vi "Write SA Pin.vi"(8 "error in (no error)":errorcluster, 10 "SA Pin":string, 11 "TDSCDMA_MODACC in":refnum<class "TDSCDMA_MODACC.lvclass">=refnum) -> (0 "error out":errorcluster, 3 "TDSCDMA_MODACC out":refnum<class "TDSCDMA_MODACC.lvclass">)   [LabVIEW 2016, in "SeqAuto Evaluations.lvlib" / "TDSCDMA_MODACC.lvclass"]
uses:
  TDSCDMA_MODACC.lvclass
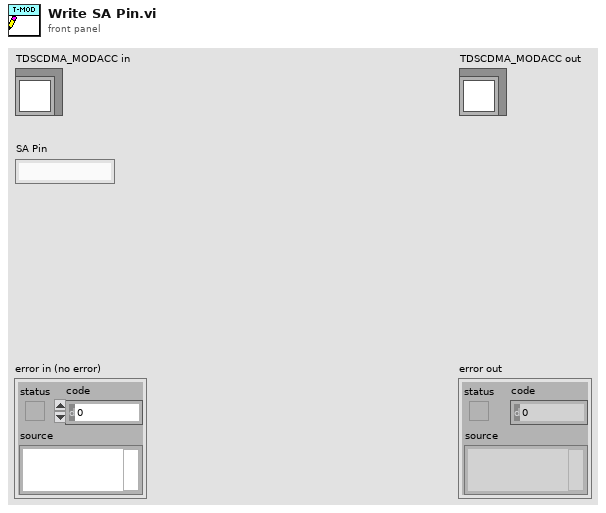
[diagram p1: front panel]
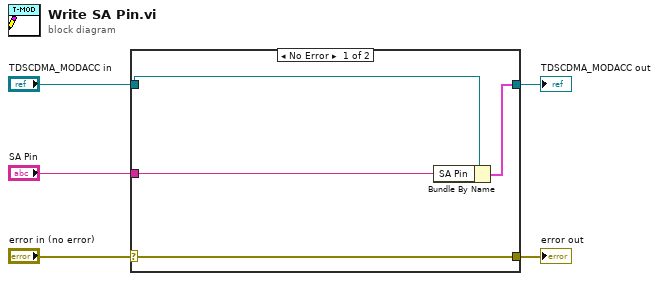
[diagram p0: block diagram]
diagram:
  n1 = case shown="No Error" "error in (no error)" {
    selector: "error in (no error)" -> [w9 w10]
    tunnel: [w9 w10] -> w4
    tunnel: [w7 w11] -> w2
    tunnel: "TDSCDMA_MODACC in" -> [w8 w11]
    tunnel: "SA Pin" -> [w6 _]
    frame No Error {
      n2 = Bundle By Name(cluster=w8, "SA Pin"=w6) -> (w7:cluster{})
    }
    frame Error {
    }
  }
  "error out" <- w4
  "TDSCDMA_MODACC out" <- w2
